vi "生成LOG波形.vi"(6 "采样":dbl, 9 "end":dbl, 10 "start":dbl, 11 "渐近线":dbl) -> (3 "波形":dbl[](array[numeric]))   [LabVIEW 2020, in "功能选择.xctl"]
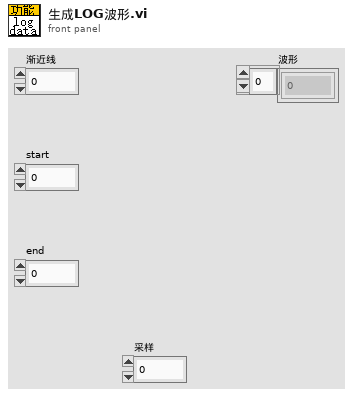
[diagram p1: front panel]
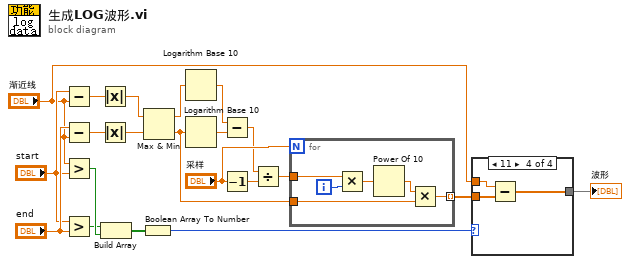
[diagram p0: block diagram]
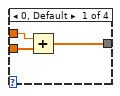
[diagram p2: hidden frame]
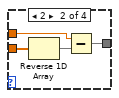
[diagram p3: hidden frame]
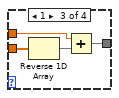
[diagram p4: hidden frame]
diagram:
  n1 = Subtract(x="start", y="渐近线") -> (x-y=w6:dbl)
  n2 = Subtract(x="end", y="渐近线") -> (x-y=w8:dbl)
  n3 = Greater?(x="渐近线", y="start") -> (0:w18:bool)
  n4 = Greater?(x="start", y="end") -> (0:w17:bool)
  n5 = Absolute Value(x=w6) -> (abs(x)=w21:dbl)
  n6 = Absolute Value(x=w8) -> (abs(x)=w11:dbl)
  n7 = Build Array(w17, w18) -> (w19:bool[])
  n8 = Boolean Array To Number(Boolean array=w19) -> (number=w20:u32)
  n9 = Max & Min(x=w21, y=w11) -> (max(x,y)=w3:dbl, min(x,y)=w2:dbl)
  n10 = Logarithm Base 10(1:w3) -> (0:w5:dbl)
  n11 = Logarithm Base 10(1:w2) -> (0:w4:dbl)
  n12 = Subtract(x=w5, y=w4) -> (x-y=w1:dbl)
  n13 = Decrement(x="采样") -> (x-1=w7:dbl)
  n14 = Divide(x=w1, y=w7) -> (x/y=w9:dbl)
  n15 = for {
    N: "采样" -> [_]
    tunnel: w2 -> [w22]
    tunnel: w9 -> [w25]
    tunnel: [w26] -> w10 mode=indexing
    i -> [w24]
    n16 = Multiply(x=w25, y=w24) -> (x*y=w27:dbl)
    n17 = Power Of 10(x=w27) -> (10^x=w23:dbl)
    n18 = Multiply(x=w23, y=w22) -> (x*y=w26:dbl)
  }
  n19 = case shown="11" w20 {
    tunnel: "渐近线" -> [w30 w34 w36 w41]
    tunnel: w10 -> [w29 w33 w37 w40]
    tunnel: [w28 w32 w35 w39] -> w14
    frame 0, Default {
      n20 = Add(x=w30, y=w29) -> (x+y=w28:dbl[])
    }
    frame 2 {
      n21 = Reverse 1D Array(array=w33) -> (reversed array=w31:dbl[])
      n22 = Subtract(x=w34, y=w31) -> (x-y=w32:dbl[])
    }
    frame 1 {
      n23 = Reverse 1D Array(array=w37) -> (reversed array=w38:dbl[])
      n24 = Add(x=w36, y=w38) -> (x+y=w35:dbl[])
    }
    frame 3 {
      n25 = Subtract(x=w41, y=w40) -> (x-y=w39:dbl[])
    }
  }
  "波形" <- w14
